vi "Add Core Dependencies.vi"(8 "error in (no error)":errorcluster, 11 "Item Ref in":T1 format="%.0x") -> (0 "error out":errorcluster, 3 "Device Ref out":T1 format="%.0x")   [LabVIEW 2020, in "DSF System Explorer.lvlib"]
uses:
  DSF System Explorer.lvlib
  <vilib>/NI VeriStand/Custom Device API/Custom Device Item Ref.ctl
  <vilib>/NI VeriStand/Custom Device API/Custom Device File Dependency.ctl
  <vilib>/NI VeriStand/Custom Device API/Path Specification.ctl
  <vilib>/NI VeriStand/Custom Device API/Path Type.ctl
  <vilib>/NI VeriStand/Custom Device API/Custom Device Supported Target.ctl
  <vilib>/NI VeriStand/Custom Device API/Custom Device API.lvlib
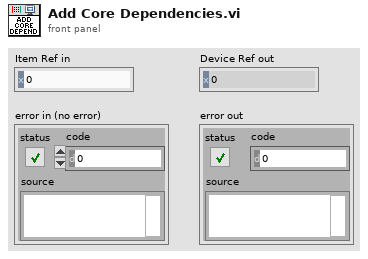
[diagram p1: front panel]
types:
  T1 = typedef "Custom Device API.lvlib/Custom Device Item Ref.ctl" = u64
  T2 = typedef "Custom Device API.lvlib/Custom Device Supported Target.ctl" = enum16{"All", "PharLap", "VxWorks", "Windows", "Linux_32_ARM", "Linux_x64", "PharLap & Windows", "PharLap & VxWorks", "VxWorks & Windows"}
  T3 = typedef "Custom Device API.lvlib/Path Type.ctl" = enum16{"Absolute", "To Base", "To Common Data Dir", "To Application Data Dir"}
  T4 = typedef "Custom Device API.lvlib/Custom Device File Dependency.ctl" = cluster{"Source":T5, "RT Destination":path, "ForceDownload?":bool, "SupportedTarget":T2, "Version":string}
  T5 = typedef "Custom Device API.lvlib/Path Specification.ctl" = cluster{"Path":path, "Type":T3}
  T6 = typedef "Custom Device API.lvlib/Custom Device Target Type.ctl" = enum16{"PharLap", "VxWorks", "Windows", "Linux_32_ARM", "Linux_x64"}
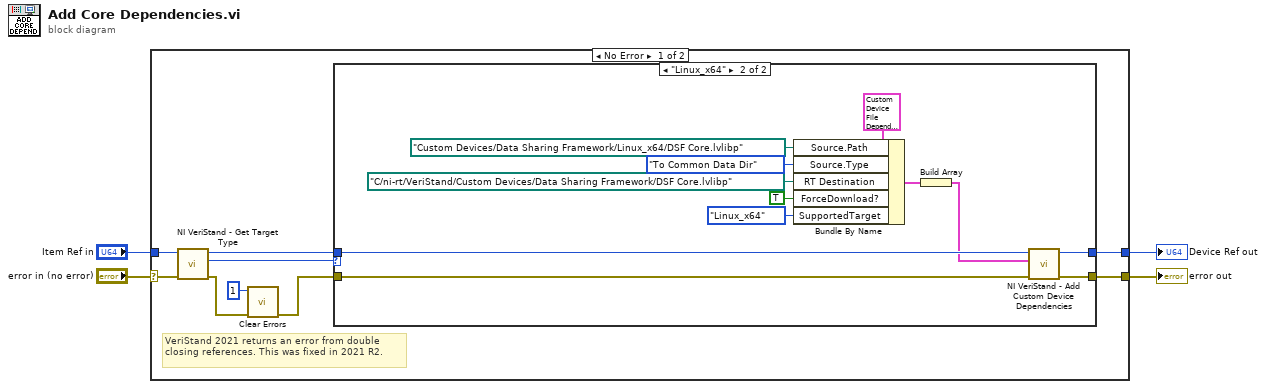
[diagram p0: block diagram]
diagram:
  n1 = case shown="No Error" "error in (no error)" {
    selector: "error in (no error)" -> [w11 w28]
    tunnel: "Item Ref in" -> [w10 w29]
    tunnel: [w9 w29] -> w2
    tunnel: [w8 w28] -> w1
    frame No Error {
      # "VeriStand 2021 returns an error from double closing references. This was fixed in 2021 R2."
      n2 = call <vilib>:"NI VeriStand - Get Target Type.vi"("error in (no error)"=w11, "Item Ref in"=w10) -> ("error out"=w6:errorcluster, "Target Type"=w13:T6, "Item Ref out"=w12:T1)  [unwired: 7 in]
      n3 = call <vilib>:"Clear Errors.vi"("error in (no error)"=w6, "specific error code to clear (0: all)"=1) -> ("error out"=w5:errorcluster)  [unwired: 4 in, 1 out]
      n4 = case shown="\"Linux_x64\"" w13 {
        tunnel: [w15 w18] -> w8
        tunnel: [w14 w17] -> w9
        tunnel: w12 -> [w14 w19]
        tunnel: w5 -> [w15 w20]
        frame "Windows", Default {
          # "Don't add dependency for Windows or unsupported target type."
        }
        frame "Linux_x64" {
          n5 = Bundle By Name(cluster=T4 {"Source"={"Path"=path "", "Type"=enum."Absolute"}, "RT Destination"=path "", "ForceDownload?"=FALSE, "SupportedTarget"=enum."PharLap", "Version"=""} ("Dependencies"), "Source.Path"=path "Custom Devices/Data Sharing Framework/Linux_x64/DSF Core.lvlibp", "Source.Type"=Path_Type."To Common Data Dir", "RT Destination"=path "C:/ni-rt/VeriStand/Custom Devices/Data Sharing Framework/DSF Core.lvlibp", "ForceDownload?"=TRUE, "SupportedTarget"=Custom_Device_Supported_Target."Linux_x64") -> (w21:T4)
          n6 = Build Array(w21) -> (w16:T4[])
          n7 = call <vilib>:"NI VeriStand - Add Custom Device Dependencies.vi"("error in (no error)"=w20, "Dependencies"=w16, "Device Ref in"=w19) -> ("error out"=w18:errorcluster, "Device Ref out"=w17:T1)  [unwired: 7 in]
        }
      }
    }
    frame Error {
    }
  }
  "Device Ref out" <- w2
  "error out" <- w1
